vi "Set Level.vi"(6 "Output Channel":T1, 8 "error in (no error)":errorcluster, 9 "Slew (V/s)":dbl, 10 "Level (V)":dbl, 11 "Inst.RP100 in":refnum<class "Inst.RP100.lvclass">) -> (0 "error out":errorcluster, 3 "Inst.RP100 out":refnum<class "Inst.RP100.lvclass">)   [LabVIEW 2019, in "Inst.RP100.lvclass"]
doc: "Set the output <b>Level</b> with <b>Slew</b> rate on the selected <b>Output Channel</b>"
uses:
  Inst.RP100.lvclass
  C:/Program Files (x86)/National Instruments/LabVIEW 2019/user.lib/LevyLab/Instrument Framework/SMOs/Instrument/Instrument.lvclass
  Typedefs/Output Channel--Enum.ctl
  Typedefs/Commands--Enum.ctl
  Typedefs/setLevel--Cluster.ctl
  <userlib>/LevyLab/Instrument Framework/SMOs/Instrument/Instrument.lvclass/Instrument.ctl
  561c9bc1-5633-4095-b2f1-945bf898e835.vi/0758c486-1f2e-4de1-be5e-979eff8f5404.vi
  561c9bc1-5633-4095-b2f1-945bf898e835.vi/0758c486-1f2e-4de1-be5e-979eff8f5404.vi/2eb98b86-8008-43ae-999f-b6359c0c8ca2.vi
  <userlib>/LevyLab/Instrument Framework/SMOs/Instrument/API/Send and Receive.vi
  561c9bc1-5633-4095-b2f1-945bf898e835.vi/0758c486-1f2e-4de1-be5e-979eff8f5404.vi/91c2f188-a780-45a8-b7b7-b95aaabe855c.vi
  <userlib>/LevyLab/Instrument Framework/SMOs/Instrument/Private/Get Client Type.vi
  561c9bc1-5633-4095-b2f1-945bf898e835.vi/0758c486-1f2e-4de1-be5e-979eff8f5404.vi/2eb98b86-8008-43ae-999f-b6359c0c8ca2.vi/af53d447-7291-46d0-a0fd-c9f53c7057a7.vi
  561c9bc1-5633-4095-b2f1-945bf898e835.vi/0758c486-1f2e-4de1-be5e-979eff8f5404.vi/2eb98b86-8008-43ae-999f-b6359c0c8ca2.vi/c6fb493c-8576-4459-999d-11640a98b674.vi
  561c9bc1-5633-4095-b2f1-945bf898e835.vi/0758c486-1f2e-4de1-be5e-979eff8f5404.vi/91c2f188-a780-45a8-b7b7-b95aaabe855c.vi/c05a6d2d-0327-479d-b366-1677f5d60a83.vi
  561c9bc1-5633-4095-b2f1-945bf898e835.vi/0758c486-1f2e-4de1-be5e-979eff8f5404.vi/91c2f188-a780-45a8-b7b7-b95aaabe855c.vi/5e05ccc7-433e-4751-9b2f-584e9c71f55e.vi
  561c9bc1-5633-4095-b2f1-945bf898e835.vi/0758c486-1f2e-4de1-be5e-979eff8f5404.vi/91c2f188-a780-45a8-b7b7-b95aaabe855c.vi/c05a6d2d-0327-479d-b366-1677f5d60a83.vi/acea0381-38c9-4709-921c-a4ba74a39ee2.vi
  561c9bc1-5633-4095-b2f1-945bf898e835.vi/0758c486-1f2e-4de1-be5e-979eff8f5404.vi/91c2f188-a780-45a8-b7b7-b95aaabe855c.vi/c05a6d2d-0327-479d-b366-1677f5d60a83.vi/01de44ba-5466-4242-8530-7722fee1969b.vi
  <userlib>/LevyLab/Instrument Framework/SMOs/Instrument/Private/Get RC Connection Status.vi
  <userlib>/LevyLab/Instrument Framework/SMOs/Instrument/API/Enum to String.vi
  <userlib>/LevyLab/Instrument Framework/SMOs/RemoteControl/API/Send and Receive.vi
  <vilib>/Utility/Data Type/Get Type Information.vi
  <vilib>/JDP Science/JSONtext/JSON text to Variant.vi
  <userlib>/LevyLab/Instrument Framework/SMOs/Instrument/API/Instrument.GetPublicEvents.vi
  <vilib>/JDP Science/JSONtext/Variant to JSON Text.vi
  <vilib>/National Instruments/GUID Generator/Guid Generator.vi
  <userlib>/LevyLab/Instrument Framework/SMOs/Instrument/API/Instrument.MessageToProcess.vi
  <userlib>/LevyLab/Instrument Framework/SMOs/Instrument/Private/Instrument.MessageFromProcess.EventStructure.vi
  <vilib>/JDP Science/JSONtext/LVClass Serializer/JSONtext LVClass Serializer.lvclass
  a747f858-0bd6-4591-9409-4ed82dc3170c.vi
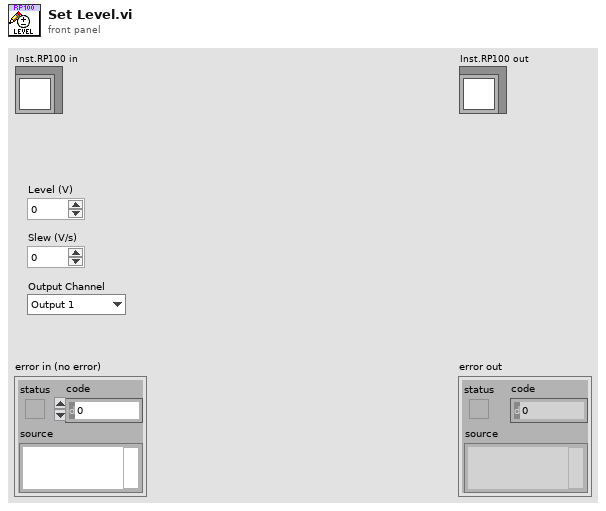
[diagram p1: front panel]
types:
  T1 = typedef "Inst.RP100.lvclass/Output Channel--Enum.ctl" = enum16{"Output 1", "Output 2"}
  T2 = typedef "Inst.RP100.lvclass/setLevel--Cluster.ctl" = cluster{"Output Channel":T1, "Level (V)":dbl, "Slew (V/s)":dbl}
  T3 = typedef "Inst.RP100.lvclass/Commands--Enum.ctl" = enum16{"setState", "setStrain", "getStrain", "setLevel", "getLevel"}
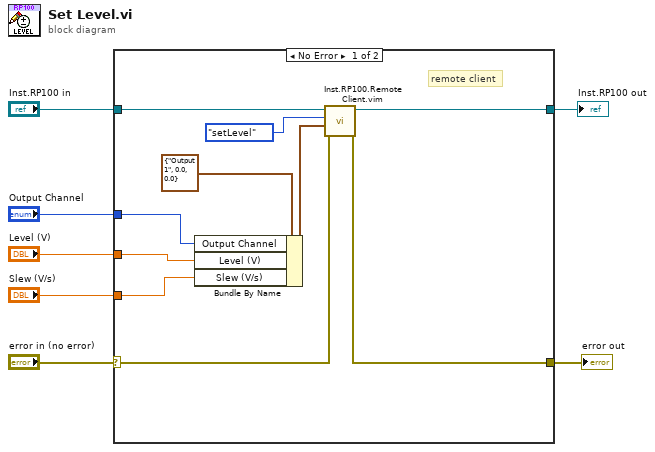
[diagram p0: block diagram]
diagram:
  n1 = case shown="No Error" "error in (no error)" {
    selector: "error in (no error)" -> [w15 w19]
    tunnel: [w14 w19] -> w6
    tunnel: "Level (V)" -> [w9 _]
    tunnel: "Inst.RP100 in" -> [w17 w18]
    tunnel: [w16 w18] -> w3
    tunnel: "Slew (V/s)" -> [w8 _]
    tunnel: "Output Channel" -> [w10 _]
    frame No Error {
      # "remote client"
      n2 = Bundle By Name(cluster=T2 {"Output Channel"=enum."Output 1", "Level (V)"=0.0, "Slew (V/s)"=0.0} ("setLevel"), "Output Channel"=w10, "Level (V)"=w9, "Slew (V/s)"=w8) -> (w11:T2)
      n3 = call "Inst.RP100.Remote Client.vim"("error in (no error)"=w15, "params"=w11, "Commands"=Commands--Enum."setLevel", "Inst.RP100 in"=w17) -> ("error out"=w14:errorcluster, "Inst.RP100 out"=w16:refnum<class "Inst.RP100.lvclass">)  [unwired: 5 in, 1 out]
    }
    frame Error {
    }
  }
  "error out" <- w6
  "Inst.RP100 out" <- w3
